vi "SR430.Get Trigger Offset us.vi"(0 "i ref in":refnum<vi>, 11 "error in (no error)":errorcluster) -> (4 "i ref out":refnum<vi>, 8 "triggerOffset [us]":dbl, 15 "error out":errorcluster)   [LabVIEW 2014, in "SR430.lvlib"]
doc: "Gets the offset (delay) of the MCS spectrum."
uses:
  SR430.lvlib
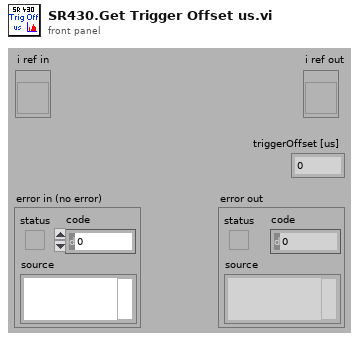
[diagram p1: front panel]
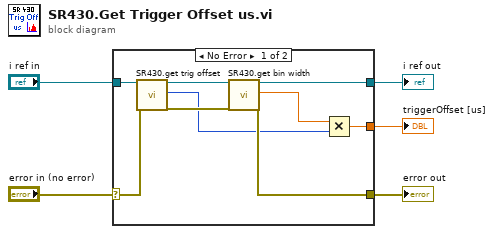
[diagram p0: block diagram]
diagram:
  n1 = case shown="No Error" "error in (no error)" {
    selector: "error in (no error)" -> [w6 w15]
    tunnel: "i ref in" -> [w14 w16]
    tunnel: [w11 w16] -> w4
    tunnel: [w10 w15] -> w3
    tunnel: [w7 _] -> w2
    frame No Error {
      n2 = call "SR430.get trig offset.vi"("i ref in"=w14, "error in (no error)"=w6) -> ("i ref out"=w12:refnum<vi>, "triggerOffset [us]"=w8:i32, "error out"=w13:errorcluster)  [unwired: 14 in, 1 out]
      n3 = call "SR430.get bin width.vi"("i ref in"=w12, "error in (no error)"=w13) -> ("i ref out"=w11:refnum<vi>, "binWidth [us]"=w9:dbl, "error out"=w10:errorcluster)  [unwired: 15 in]
      n4 = Multiply(x=w9, y=w8) -> (x*y=w7:dbl)
    }
    frame Error {
    }
  }
  "i ref out" <- w4
  "error out" <- w3
  "triggerOffset [us]" <- w2
